vi "MGI Search Sorted.vi"(8 "Search String":string, 10 "Sorted Strings":string[](array[string])) -> (0 "Found":bool, 1 "Closest Match":i32, 2 "Result":string, 3 "Where to Insert":i32)   [LabVIEW 2016]
doc: "Search a sorted list of strings using a binary search. Additional outputs are helpful in maintaining the sorted list.\n\nAuthored by Shawn Walpole\nsupport@mooregoodideas.com\nwww.mooregoodideas.com\n\nCopyright (c) 2010, Moore Good Ideas, Inc.\n\nAll rights reserved.\n\nRedistribution and use in source and binary forms, with or without modification, are permitted provided that the following conditions are met:\n\n * Redistributions of source code must retain the above copyright notice, this list of conditions and the following disclaimer.\n * Redistributions in binary form must reproduce the above copyright notice, this list of conditions and the following disclaimer in the documentation and/or other materials provided with the distribution.\n * Neither the name of Moore Good Ideas, Inc. nor the names of its contributors may be used to endorse or promote products derived from this software without specific prior written permission.\n\nTHIS SOFTWARE IS PROVIDED BY THE COPYRIGHT HOLDERS AND CONTRIBUTORS \"AS IS\" AND ANY EXPRESS OR IMPLIED WARRANTIES, INCLUDING, BUT NOT LIMITED TO, THE IMPLIED WARRANTIES OF MERCHANTABILITY AND FITNESS FOR A PARTICULAR PURPOSE ARE DISCLAIMED. IN NO EVENT SHALL THE COPYRIGHT OWNER OR CONTRIBUTORS BE LIABLE FOR ANY DIRECT, INDIRECT, INCIDENTAL, SPECIAL, EXEMPLARY, OR CONSEQUENTIAL DAMAGES (INCLUDING, BUT NOT LIMITED TO, PROCUREMENT OF SUBSTITUTE GOODS OR SERVICES; LOSS OF USE, DATA, OR PROFITS; OR BUSINESS INTERRUPTION) HOWEVER CAUSED AND ON ANY THEORY OF LIABILITY, WHETHER IN CONTRACT, STRICT LIABILITY, OR TORT (INCLUDING NEGLIGENCE OR OTHERWISE) ARISING IN ANY WAY OUT OF THE USE OF THIS SOFTWARE, EVEN IF ADVISED OF THE POSSIBILITY OF SUCH DAMAGE."
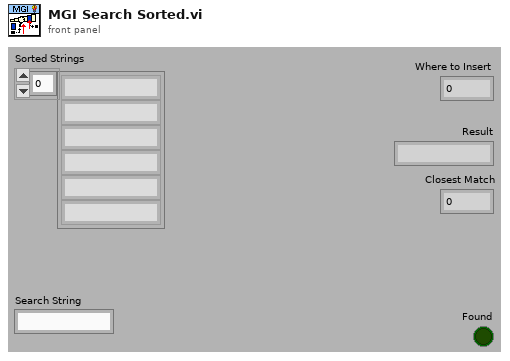
[diagram p1: front panel]
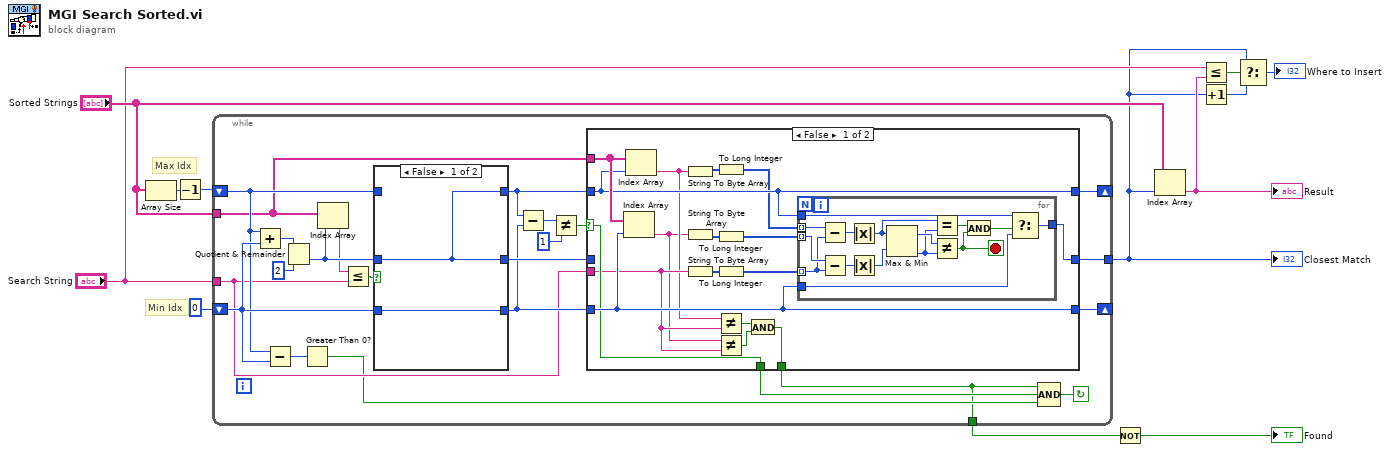
[diagram p0: block diagram]
diagram:
  # "Min Idx"
  # "Max Idx"
  n1 = Array Size(array="Sorted Strings") -> (size(s)=w3:i32)
  n2 = Decrement(x=w3) -> (x-1=w11:i32)
  n3 = while {
    tunnel: "Sorted Strings" -> [w17]
    tunnel: "Search String" -> [w16]
    shift-right: [w24] -> _
    shift-left: w11 -> [w29]
    shift-right: [w26] -> _
    shift-left: 0 ("y") -> [w30]
    tunnel: [w25] -> w4
    tunnel: [w13] -> w1
    stop <- w35 continue-if-true
    n4 = Add(x=w29, y=w30) -> (x+y=w33:i32)
    n5 = Subtract(x=w29, y=w30) -> (x-y=w27:i32)
    n6 = Quotient & Remainder(x=w33, y=2) -> (floor(x/y)=w31:i32)  [unwired: 1 out]
    n7 = Greater Than 0?(x=w27) -> (x > 0?=w15:bool)
    n8 = Index Array(array=w17, index=w31) -> (element=w28:string)
    n9 = Less Or Equal?(x=w28, y=w16) -> (x <= y?=w34:bool)
    n10 = case shown="False" w34 {
      tunnel: w31 -> [w37 w38]
      tunnel: w30 -> [w36 _]
      tunnel: w29 -> [_ w39]
      tunnel: [w36 w38] -> w21
      tunnel: [w37 w39] -> w22
      tunnel: [w37 w38] -> w23
      frame False {
      }
      frame True {
      }
    }
    n11 = Subtract(x=w22, y=w21) -> (x-y=w20:i32)
    n12 = Not Equal?(x=w20, y=1) -> (x != y?=w18:bool)
    n13 = case shown="False" w18 {
      selector: w18 -> [w43 w72]
      tunnel: [w48 w75] -> w26
      tunnel: w21 -> [w48 w75]
      tunnel: [w47 w74] -> w25
      tunnel: w23 -> [_ w74]
      tunnel: [w52 w73] -> w24
      tunnel: w22 -> [w52 w73]
      tunnel: w17 -> [w56 _]
      tunnel: w16 -> [w42 _]
      tunnel: [w43 w72] -> w14
      tunnel: [w44 w72] -> w13
      frame False {
        n14 = Index Array(array=w56, index=w48) -> (element=w40:string)
        n15 = Index Array(array=w56, index=w52) -> (element=w41:string)
        n16 = String To Byte Array(string=w41) -> (unsigned byte array=w55:u8[])
        n17 = String To Byte Array(string=w40) -> (unsigned byte array=w54:u8[])
        n18 = String To Byte Array(string=w42) -> (unsigned byte array=w53:u8[])
        n19 = To Long Integer(number=w55) -> (32bit integer=w51:i32[])
        n20 = To Long Integer(number=w54) -> (32bit integer=w50:i32[])
        n21 = To Long Integer(number=w53) -> (32bit integer=w49:i32[])
        n22 = Not Equal?(x=w41, y=w42) -> (x != y?=w46:bool)
        n23 = Not Equal?(x=w40, y=w42) -> (x != y?=w45:bool)
        n24 = And(x=w46, y=w45) -> (x .and. y?=w44:bool)
        n25 = for {
          tunnel: w52 -> [w64]
          tunnel: w51 -> [w71] mode=indexing
          tunnel: w50 -> [w70] mode=indexing
          tunnel: w49 -> [w69] mode=indexing
          tunnel: w48 -> [w63]
          tunnel: [w62] -> w47
          stop <- w57 stop-if-true
          n26 = Subtract(x=w71, y=w69) -> (x-y=w68:i32)
          n27 = Subtract(x=w70, y=w69) -> (x-y=w67:i32)
          n28 = Absolute Value(x=w68) -> (abs(x)=w65:i32)
          n29 = Absolute Value(x=w67) -> (abs(x)=w66:i32)
          n30 = Max & Min(x=w65, y=w66) -> (max(x,y)=w60:i32, min(x,y)=w59:i32)
          n31 = Equal?(x=w65, y=w59) -> (x = y?=w61:bool)
          n32 = Not Equal?(x=w60, y=w59) -> (x != y?=w57:bool)
          n33 = And(x=w61, y=w57) -> (x .and. y?=w58:bool)
          n34 = Select(t=w64, s=w58, f=w63) -> (s? t:f=w62:i32)
        }
      }
      frame True {
      }
    }
    n35 = Compound Arithmetic op=AND(w13, w14, w15) -> (w35:bool)
  }
  "Closest Match" <- w4
  n36 = Not(x=w1) -> (.not. x?=→"Found":bool)
  n37 = Index Array(array="Sorted Strings", index=w4) -> (element=w7:string)
  "Result" <- w7
  n38 = Less Or Equal?(x="Search String", y=w7) -> (x <= y?=w6:bool)
  n39 = Increment(x=w4) -> (x+1=w5:i32)
  n40 = Select(t=w4, s=w6, f=w5) -> (s? t:f=→"Where to Insert":i32)
